vi "Arm Speed Logic.vi"(10 "Arm Current":dbl, 11 "Arm Set":dbl) -> (3 "Arm Motor":dbl)   [LabVIEW 2012]
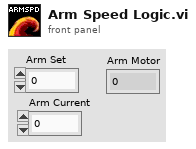
[diagram p1: front panel]
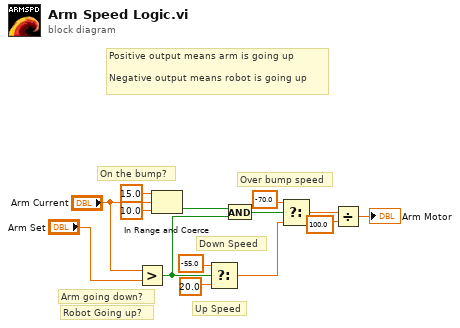
[diagram p0: block diagram]
diagram:
  # "Positive output means arm is going up\n\nNegative output means robot is going up"
  # "Arm going down?"
  # "Robot Going up?"
  # "On the bump?"
  # "Over bump speed"
  # "Up Speed"
  # "Down Speed"
  n1 = Greater?(x="Arm Current", y="Arm Set") -> (0:w1:bool)
  n2 = In Range and Coerce(upper limit=15.0, x="Arm Current", lower limit=10.0) -> (In Range?=w7:bool)  [unwired: 1 out]
  n3 = Select(t=-55.0, s=w1, f=20.0) -> (s? t:f=w2:dbl)
  n4 = And(x=w7, y=w1) -> (x .and. y?=w12:bool)
  n5 = Select(t=-70.0, s=w12, f=w2) -> (s? t:f=w9:dbl)
  n6 = Divide(x=w9, y=100.0) -> (x/y=→"Arm Motor":dbl)
